vi "Strip Word.vi"(8 "error in (no error)":errorcluster, 10 "String":string, 11 "ProtoParser in":refnum<class "ProtoParser.lvclass">) -> (0 "error out":errorcluster, 1 "Word":string, 2 "Remaining":string, 3 "ProtoParser out":refnum<class "ProtoParser.lvclass">)   [LabVIEW 2024, in "LV-Protoc.lvlib" / "ProtoParser.lvclass"]
uses:
  ProtoParser.lvclass
  ProtoParser.lvclass/ProtoParser.ctl
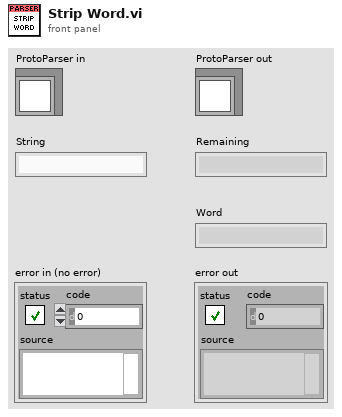
[diagram p1: front panel]
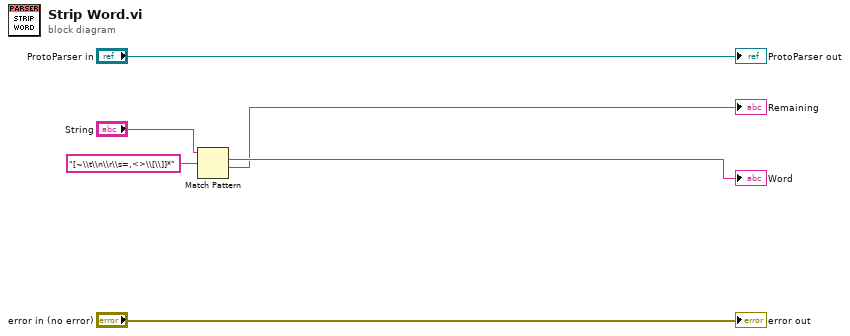
[diagram p0: block diagram]
diagram:
  n1 = Match Pattern(string="String", regular expression="[~\\t\\n\\r\\s=,<>\\[\\]]*") -> (match substring=→"Word":string, after substring=→"Remaining":string)  [unwired: 1 in, 2 out]
  "error out" <- "error in (no error)"
  "ProtoParser out" <- "ProtoParser in"
